vi "_isExpectedDataPluginCell.vi"(6 "Column":i32=3, 8 "error in (no error)":errorcluster, 9 "Row":i32, 10 "Coords":T1, 11 "MulticolumnListbox":refnum<vi>) -> (0 "error out":errorcluster, 3 "result":bool)   [LabVIEW 2020]
uses:
  <vilib>/Utility/miscctls.llb/LVPoint32TypeDef.ctl
  <vilib>/Utility/miscctls.llb/LVRowAndColumnTypeDef.ctl
  <vilib>/Utility/miscctls.llb/LVRowAndColumnUnsignedTypeDef.ctl
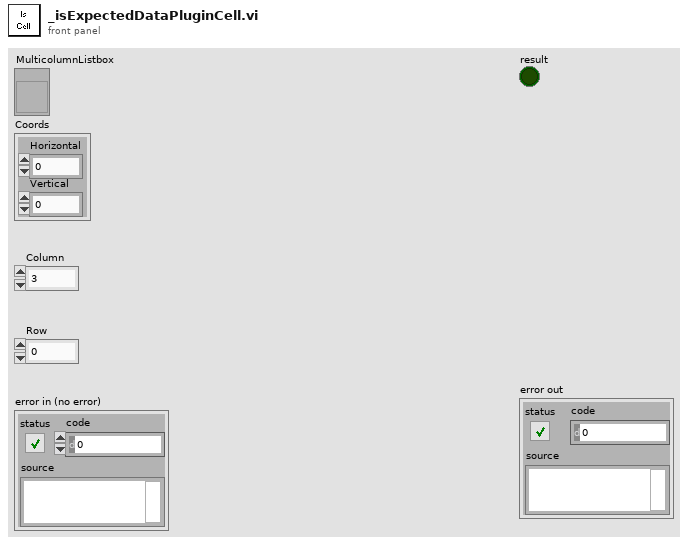
[diagram p1: front panel]
types:
  T1 = typedef "LVPoint32TypeDef.ctl" = cluster{"Horizontal":i32, "Vertical":i32}
  T2 = typedef "LVRowAndColumnTypeDef.ctl" = cluster{"Row":i32, "Column":i32}
  T3 = typedef "LVRowAndColumnUnsignedTypeDef.ctl" = cluster{"Row":u32, "Column":u32}
  T4 = typedef "LVPositionTypeDef.ctl" = cluster{"Left":i32, "Top":i32}
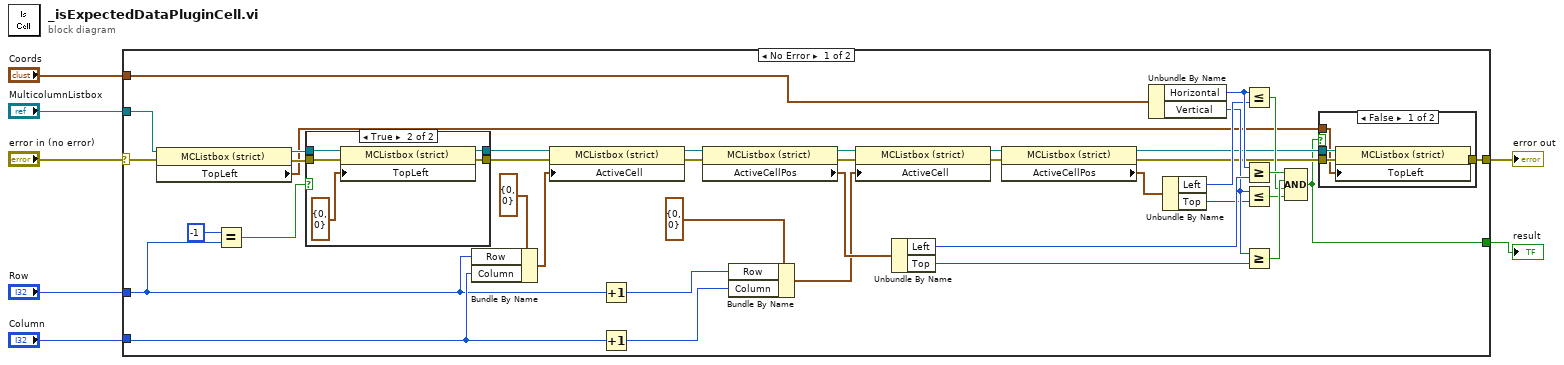
[diagram p0: block diagram]
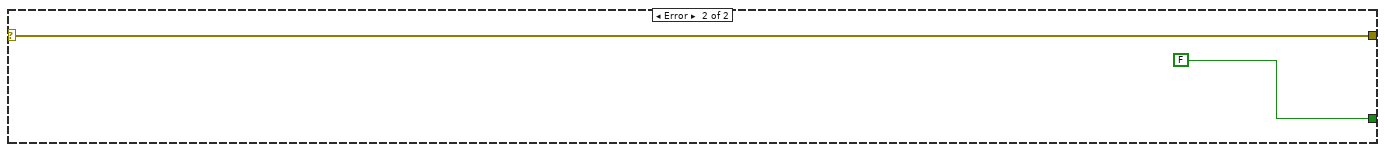
[diagram p4: hidden frame]
diagram:
  n1 = case shown="No Error" "error in (no error)" {
    selector: "error in (no error)" -> [w15 w61]
    tunnel: "Coords" -> [w47 _]
    tunnel: [w8 FALSE] -> w6
    tunnel: "MulticolumnListbox" -> [w16 _]
    tunnel: "Row" -> [w19 _]
    tunnel: "Column" -> [w33 _]
    tunnel: [w11 w61] -> w2
    frame No Error {
      n2 = property class="MCListbox (strict)"(reference=w16, error in=w15) -> (reference out=w14:refnum<vi>, error out=w13:errorcluster, "TopLeft"=w9:T3)
      n3 = Equal?(x=-1, y=w19) -> (x = y?=w18:bool)
      n4 = case shown="True" w18 {
        tunnel: [w53 w59] -> w21
        tunnel: [w54 w58] -> w20
        tunnel: w13 -> [w53 w57]
        tunnel: w14 -> [w54 w56]
        frame False {
        }
        frame True {
          n5 = property class="MCListbox (strict)"(reference=w56, error in=w57, "TopLeft"=T3 {"Row"=0, "Column"=0} ("Top Left Visible Cell")) -> (reference out=w58:refnum<vi>, error out=w59:errorcluster)
        }
      }
      n6 = Bundle By Name(cluster=T2 {"Row"=0, "Column"=0} ("Active Cell:Active Cell"), "Row"=w19, "Column"=w33) -> (w22:T2)
      n7 = property class="MCListbox (strict)"(reference=w20, error in=w21, "ActiveCell"=w22) -> (reference out=w36:refnum<vi>, error out=w35:errorcluster)
      n8 = Increment(x=w19) -> (x+1=w27:i32)
      n9 = Increment(x=w33) -> (x+1=w25:i32)
      n10 = property class="MCListbox (strict)"(reference=w36, error in=w35) -> (reference out=w28:refnum<vi>, error out=w29:errorcluster, "ActiveCellPos"=w32:T4)
      n11 = Bundle By Name(cluster=T2 {"Row"=0, "Column"=0} ("Active Cell:Active Cell"), "Row"=w27, "Column"=w25) -> (w24:T2)
      n12 = property class="MCListbox (strict)"(reference=w28, error in=w29, "ActiveCell"=w24) -> (reference out=w31:refnum<vi>, error out=w30:errorcluster)
      n13 = Unbundle By Name(w32) -> ("Left"=w46:i32, "Top"=w43:i32)
      n14 = property class="MCListbox (strict)"(reference=w31, error in=w30) -> (reference out=w10:refnum<vi>, error out=w12:errorcluster, "ActiveCellPos"=w23:T4)
      n15 = Unbundle By Name(w47) -> ("Horizontal"=w45:i32, "Vertical"=w42:i32)
      n16 = Unbundle By Name(w23) -> ("Left"=w44:i32, "Top"=w37:i32)
      n17 = Less Or Equal?(x=w45, y=w44) -> (x <= y?=w39:bool)
      n18 = Greater Or Equal?(x=w45, y=w46) -> (x >= y?=w41:bool)
      n19 = Less Or Equal?(x=w42, y=w37) -> (x <= y?=w38:bool)
      n20 = Greater Or Equal?(x=w42, y=w43) -> (x >= y?=w40:bool)
      n21 = Compound Arithmetic op=AND(w41, w40, w39, w38) -> (w8:bool)
      n22 = case shown="False" w8 {
        tunnel: w12 -> [w51 w52]
        tunnel: [w50 w52] -> w11
        tunnel: w10 -> [w49 _]
        tunnel: w9 -> [w48 _]
        frame False {
          n23 = property class="MCListbox (strict)"(reference=w49, error in=w51, "TopLeft"=w48) -> (error out=w50:errorcluster)  [unwired: 1 out]
        }
        frame True {
        }
      }
    }
    frame Error {
    }
  }
  "result" <- w6
  "error out" <- w2
